vi "SmartMotor_parse status word zero bits.vi"(8 "error in (no error)":errorcluster, 11 "SW0 in":dbl) -> (0 "error out":errorcluster, 1 "Motor OFF":bool, 2 "InTrajMotion":bool, 3 "SW0 Bits out":T1, 5 "Negative Limit":bool, 7 "Positive Limit":bool)   [LabVIEW 2020]
doc: "Developed by Kevin Thompson\nkevin@thompsonengineering.net\n\nCopyright 2018-2020\nThompson Engineering, LLC"
uses:
  TD SW0 Bits_cluster.ctl
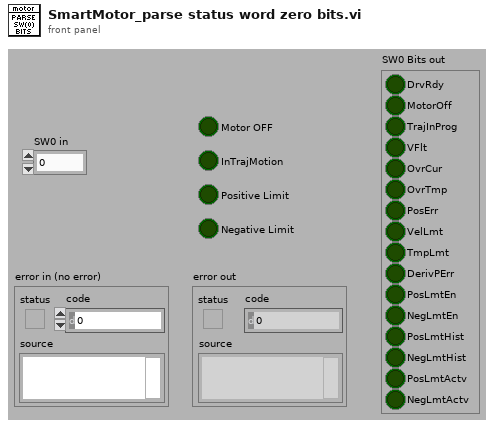
[diagram p1: front panel]
types:
  T1 = typedef "TD SW0 Bits_cluster.ctl" = cluster{"DrvRdy":bool, "MotorOff":bool, "TrajInProg":bool, "VFlt":bool, "OvrCur":bool, "OvrTmp":bool, "PosErr":bool, "VelLmt":bool, "TmpLmt":bool, "DerivPErr":bool, "PosLmtEn":bool, "NegLmtEn":bool, "PosLmtHist":bool, "NegLmtHist":bool, "PosLmtActv":bool, "NegLmtActv":bool}
  T2 = cluster{"Boolean array[0]":bool, "Boolean array[1]":bool, "Boolean array[2]":bool, "Boolean array[3]":bool, "Boolean array[4]":bool, "Boolean array[5]":bool, "Boolean array[6]":bool, "Boolean array[7]":bool, "Boolean array[8]":bool, "Boolean array[9]":bool, "Boolean array[10]":bool, "Boolean array[11]":bool, "Boolean array[12]":bool, "Boolean array[13]":bool, "Boolean array[14]":bool, "Boolean array[15]":bool}
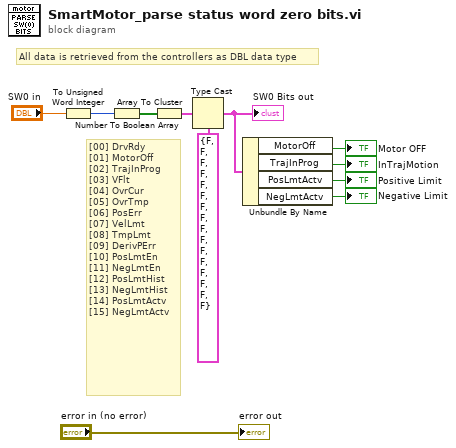
[diagram p0: block diagram]
diagram:
  # "[00] DrvRdy\n[01] MotorOff\n[02] TrajInProg\n[03] VFlt\n[04] OvrCur\n[05] OvrTmp\n[06] PosErr\n[07] VelLmt\n[08] TmpLmt\n[09] DerivPErr\n[10] PosLmtEn\n[11] NegLmtEn\n[12] PosLmtHist\n[13] NegLmtHist\n[14] PosLmtActv\n[15] NegLmtActv"
  # "All data is retrieved from the controllers as DBL data type"
  n1 = To Unsigned Word Integer(number="SW0 in") -> (unsigned 16bit integer=w10:u16)
  n2 = Number To Boolean Array(number=w10) -> (Boolean array=w9:bool[])
  n3 = Array To Cluster(array=w9) -> (cluster=w7:T2)
  n4 = Type Cast(type=T1 {"DrvRdy"=FALSE, "MotorOff"=FALSE, "TrajInProg"=FALSE, "VFlt"=FALSE, "OvrCur"=FALSE, "OvrTmp"=FALSE, "PosErr"=FALSE, "VelLmt"=FALSE, "TmpLmt"=FALSE, "DerivPErr"=FALSE, "PosLmtEn"=FALSE, "NegLmtEn"=FALSE, "PosLmtHist"=FALSE, "NegLmtHist"=FALSE, "PosLmtActv"=FALSE, "NegLmtActv"=FALSE} ("SW0_Bits"), x=w7) -> (*(type *) &x=w5:T1)
  "SW0 Bits out" <- w5
  n5 = Unbundle By Name(w5) -> ("MotorOff"=→"Motor OFF":bool, "TrajInProg"=→"InTrajMotion":bool, "PosLmtActv"=→"Positive Limit":bool, "NegLmtActv"=→"Negative Limit":bool)
  "error out" <- "error in (no error)"
